vi "Htr Const Calc.vi"(0 "Htr Set V (V)":dbl, 1 "Htr Const Mode":bool, 2 "Htr Set P (W)":dbl, 3 "Htr V_Lim (V)":dbl, 4 "Htr Res (ohms)":dbl) -> (5 "Htr Set (%)":dbl)   [LabVIEW 2013]
panel:
  # "TRUE = Const P mode\nFALSE = Const V mode"
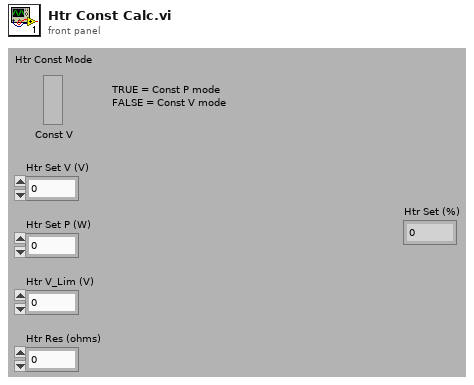
[diagram p1: front panel]
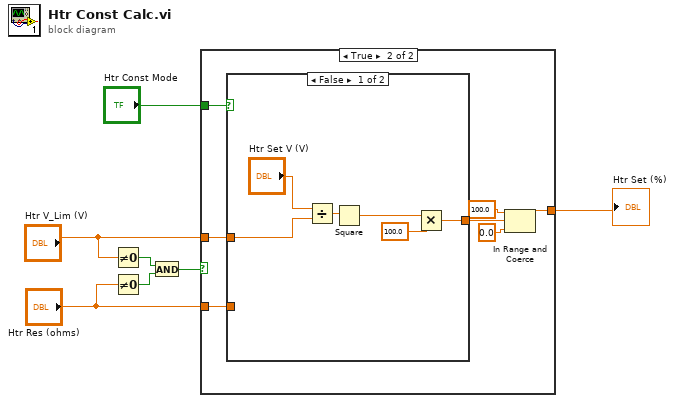
[diagram p0: block diagram]
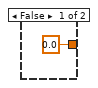
[diagram p2: hidden frame]
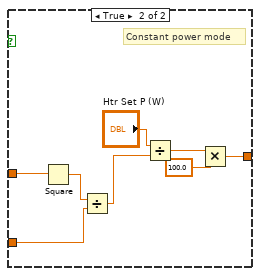
[diagram p3: hidden frame]
diagram:
  n1 = Not Equal To 0?(x="Htr V_Lim (V)") -> (x != 0?=w2:bool)
  n2 = Not Equal To 0?(x="Htr Res (ohms)") -> (x != 0?=w3:bool)
  n3 = And(x=w2, y=w3) -> (x .and. y?=w6:bool)
  n4 = case shown="True" w6 {
    tunnel: "Htr V_Lim (V)" -> [_ w15]
    tunnel: "Htr Res (ohms)" -> [_ w14]
    tunnel: [0.0 ("upper limit") w9] -> w7
    tunnel: "Htr Const Mode" -> [_ w13]
    frame False {
    }
    frame True {
      n5 = case shown="False" w13 {
        tunnel: w15 -> [w20 w28]
        tunnel: w14 -> [_ w25]
        tunnel: [w16 w22] -> w10
        frame False {
          n6 = Divide(x="Htr Set V (V)", y=w20) -> (x/y=w19:dbl)
          n7 = Square(x=w19) -> (x^2=w18:dbl)
          n8 = Multiply(x=w18, y=100.0) -> (x*y=w16:dbl)
        }
        frame True {
          # "Constant power mode"
          n9 = Square(x=w28) -> (x^2=w29:dbl)
          n10 = Divide(x=w29, y=w25) -> (x/y=w27:dbl)
          n11 = Divide(x="Htr Set P (W)", y=w27) -> (x/y=w23:dbl)
          n12 = Multiply(x=w23, y=100.0) -> (x*y=w22:dbl)
        }
      }
      n13 = In Range and Coerce(upper limit=100.0, x=w10, lower limit=0.0) -> (coerced(x)=w9:dbl)  [unwired: 1 out]
    }
  }
  "Htr Set (%)" <- w7
